vi "Dispose DataColumn.vi"(8 "error in (no error)":errorcluster caption="错误输入（无错误）", 11 "Data Column 输入":refnum<class "Data Column.lvclass"> caption="DNL_LabVIEW Object in") -> (0 "error out":errorcluster caption="错误输出", 3 "Data Column 输出":refnum<class "Data Column.lvclass"> caption="DNL_LabVIEW Object out")   [LabVIEW 2012, in "Data Grid VIEW.lvlib" / "Data Column.lvclass"]
uses:
  Data Column.lvclass
  Data Column.lvclass/Data Column.ctl
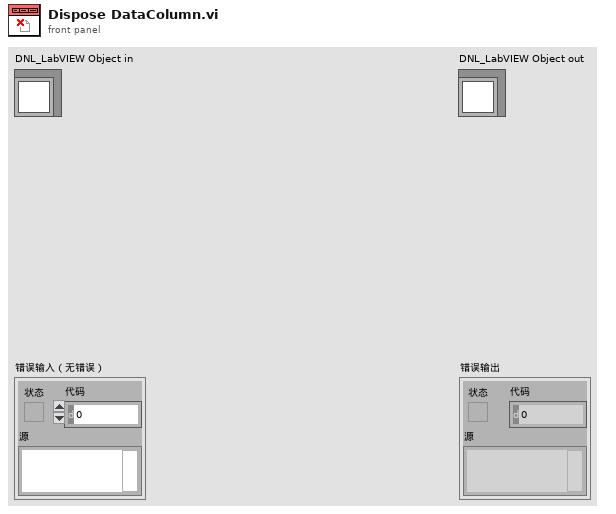
[diagram p1: front panel]
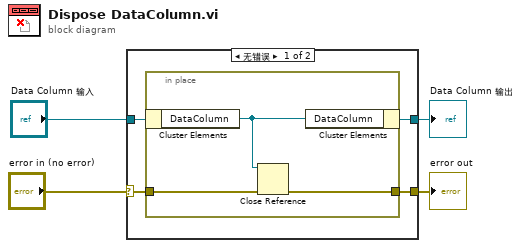
[diagram p0: block diagram]
diagram:
  n1 = case shown="无错误" "error in (no error)" {
    selector: "error in (no error)" -> [w7 w13]
    tunnel: [w6 w13] -> w3
    tunnel: [w5 w12] -> w1
    tunnel: "Data Column 输入" -> [w8 w12]
    frame No Error {
      n2 = in-place {
        in-place-border: w7 -> [w11]
        in-place-border: [w10] -> w6
        n3 = in-place-cluster #1(w8) -> ("DataColumn"=w9:refnum<k24>)
        n4 = Close Reference(reference=w9, error in (no error)=w11) -> (error out=w10:errorcluster)
        n5 = in-place-cluster #1("DataColumn"=w9) -> (w5:refnum<class "Data Column.lvclass">)
      }
    }
    frame Error {
    }
  }
  "error out" <- w3
  "Data Column 输出" <- w1
